vi "Find Build Spec Destinations.vi"(8 "error in":errorcluster, 11 "consumer data":T1) -> (0 "error out":errorcluster, 1 "template xml file":string, 2 "template built directory":string, 3 "consumer data out":T1)   [LabVIEW 2020, in "Template Tool.lvlib"]
uses:
  Template Tool.lvlib
  Consumer Data.ctl
  Project Build Specs.ctl
  <vilib>/regexp/Match Regular Expression.xnode
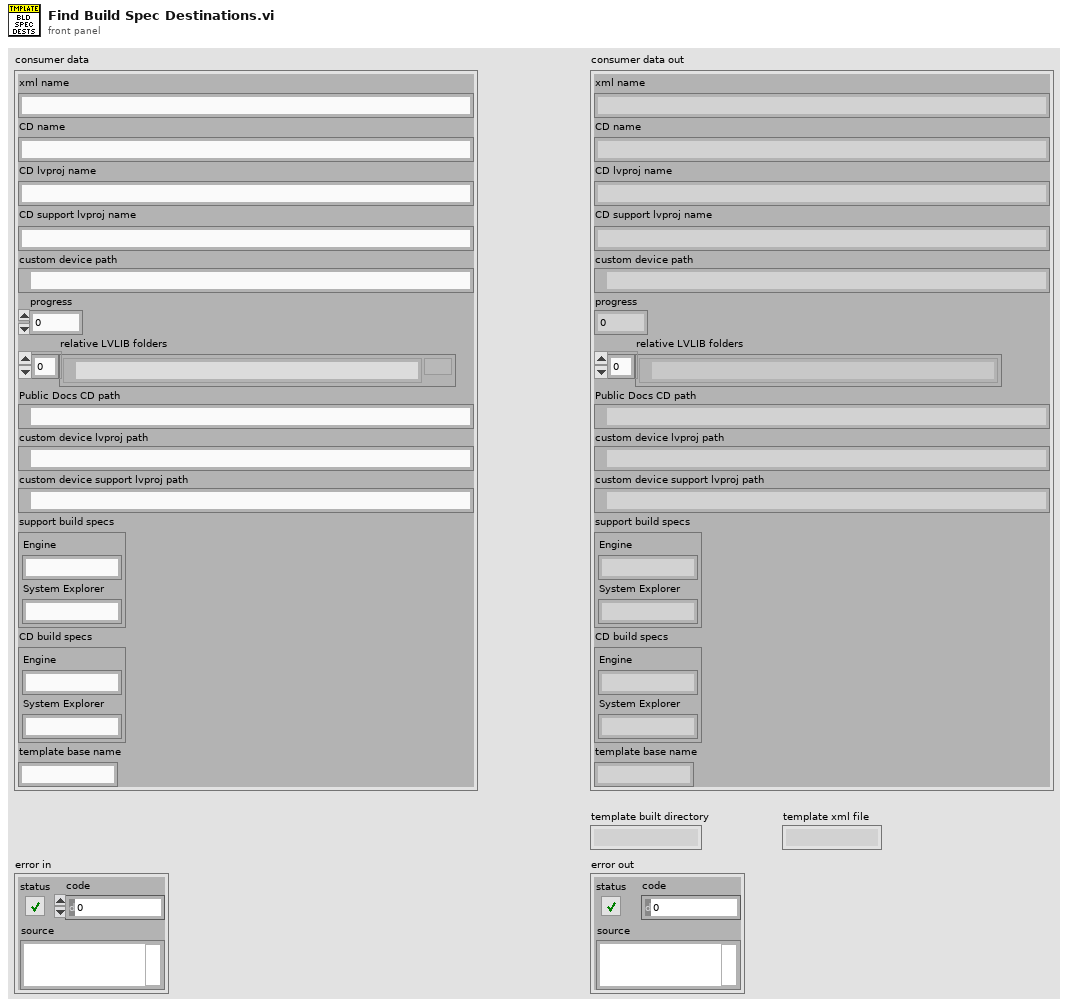
[diagram p1: front panel]
types:
  T1 = typedef "Template Tool.lvlib/Consumer Data.ctl" = cluster{"xml name":string, "CD name":string, "CD lvproj name":string, "CD support lvproj name":string, "custom device path":path, "progress":u8, "relative LVLIB folders":path[], "Public Docs CD path":path, "custom device lvproj path":path, "custom device support lvproj path":path, "support build specs":T2, "CD build specs":T2, "template base name":string}
  T2 = typedef "Template Tool.lvlib/Project Build Specs.ctl" = cluster{"Engine":string, "System Explorer":string}
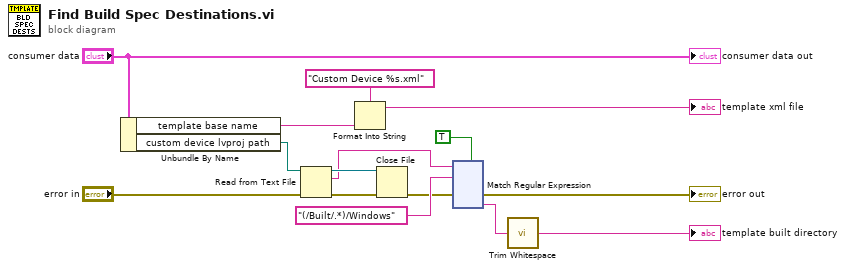
[diagram p0: block diagram]
diagram:
  n1 = Unbundle By Name("consumer data") -> ("template base name"=w2:string, "custom device lvproj path"=w4:path)
  n2 = Read from Text File(file (use dialog)=w4, error in="error in") -> (refnum out=w13:refnum<file>, text=w10:string, error out=w14:errorcluster)  [unwired: 2 in, 1 out]
  n3 = Format Into String(format string="Custom Device %s.xml", w2) -> (resulting string=→"template xml file":string)  [unwired: 2 in, 1 out]
  n4 = Close File(refnum=w13, error in=w14) -> (error out=w8:errorcluster)  [unwired: 1 out]
  n5 = xnode "Match Regular Expression"("input string"=w10, "regular expression"="(/Built/.*)/Windows" ("search string"), "error in"=w8, "multiline? (F)"=TRUE) -> ("error out"=→"error out":errorcluster, "submatch 1"=w11:string)  [unwired: 2 in, 4 out]
  n6 = call <vilib>:"Trim Whitespace.vi"("string"=w11) -> ("trimmed string"=→"template built directory":string)  [unwired: 1 in]
  "consumer data out" <- "consumer data"
